vi "Calc.vi"() -> ()   [LabVIEW 2021]
panel:
  in  "Equals":bool
  in  "Operation":string(combo)
  out "Output":dbl
  in  "Input 2":dbl
  in  "Input 1":dbl
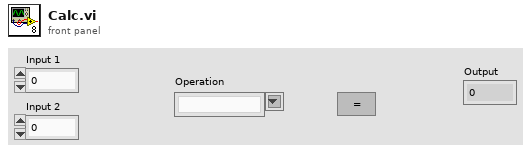
[diagram p1: front panel]
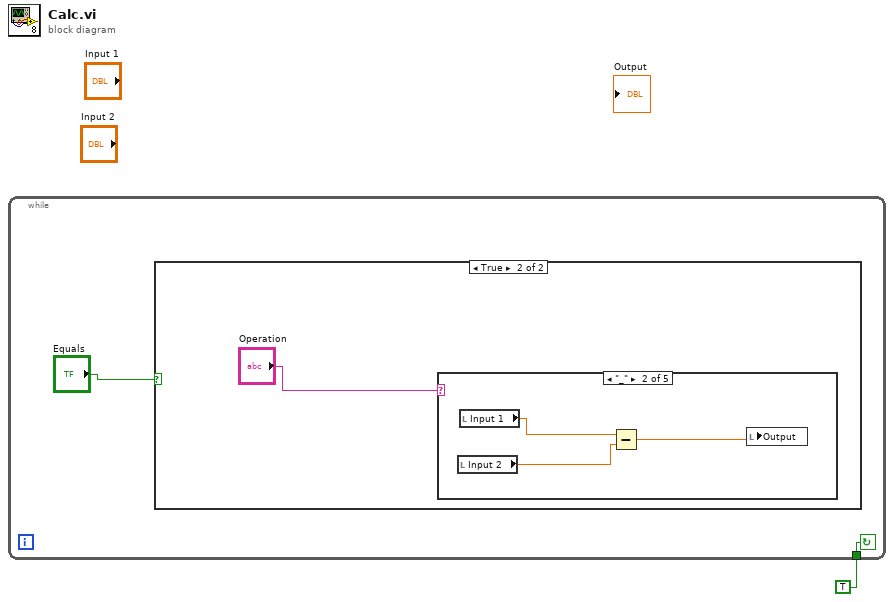
[diagram p0: block diagram]
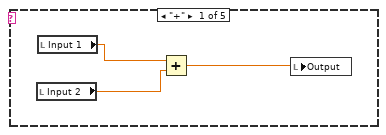
[diagram p3: hidden frame]
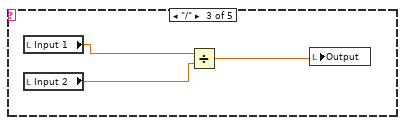
[diagram p4: hidden frame]
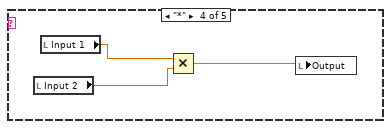
[diagram p5: hidden frame]
diagram:
  n1 = while {
    tunnel: TRUE -> [w2]
    stop <- w2 continue-if-true
    n2 = case shown="True" "Equals" {
      frame False {
      }
      frame True {
        n3 = case shown="\"_\"" "Operation" {
          frame "+" {
            n4 = local read "Input 2"() -> (w6:dbl)
            n5 = local read "Input 1"() -> (w7:dbl)
            n6 = Add(x=w7, y=w6) -> (x+y=w5:dbl)
            n7 = local write "Output"(w5) -> ()
          }
          frame "_" {
            n8 = local read "Input 2"() -> (w9:dbl)
            n9 = local read "Input 1"() -> (w10:dbl)
            n10 = Subtract(x=w10, y=w9) -> (x-y=w8:dbl)
            n11 = local write "Output"(w8) -> ()
          }
          frame "/" {
            n12 = local read "Input 1"() -> (w13:dbl)
            n13 = local read "Input 2"() -> (w12:dbl)
            n14 = Divide(x=w13, y=w12) -> (x/y=w11:dbl)
            n15 = local write "Output"(w11) -> ()
          }
          frame "*" {
            n16 = local read "Input 2"() -> (w15:dbl)
            n17 = local read "Input 1"() -> (w16:dbl)
            n18 = Multiply(x=w16, y=w15) -> (x*y=w14:dbl)
            n19 = local write "Output"(w14) -> ()
          }
          frame Default {
          }
        }
      }
    }
  }
